vi "FieldPlaneRotation.vi"(8 "Bv (T)":dbl, 9 "Bu (T)":dbl, 10 "AlfaY (rad)":dbl, 11 "AlfaX (rad)":dbl) -> (1 "Bz (T)":dbl, 2 "By (T)":dbl, 3 "Bx (T)":dbl)   [LabVIEW 2020]
uses:
  <vilib>/imath/engines/lvmath2/RunTimeEngine/ArithmeticOperatorToken/NIMS_ArithmeticOperator_multmx-internal.vi
  <instcachedir>/0/NIMS_ArithmeticOperator_multmx-internal_B44B9A6937C8407A9A8862E3F2935EB3.lvgen/NIMS_ArithmeticOperator_multmx-internal_B44B9A6937C8407A9A8862E3F2935EB3_004.vi
  <vilib>/imathl/engines/lvmath/Functions/Error Handling/Create Error.vi
  <vilib>/imath/engines/lvmath2/RunTimeEngine/ArithmeticOperatorToken/NIMS_ArithmeticOperator_multmx(M,CV)-internal.vi
  <instcachedir>/0/NIMS_ArithmeticOperator_multmx(M,CV)-internal_19A14CC5BE0A4D31BE1E94A2E998D8C3.lvgen/NIMS_ArithmeticOperator_multmx(M,CV)-internal_19A14CC5BE0A4D31BE1E94A2E998D8C3_001.vi
  <vilib>/imath/engines/lvmath2/RunTimeEngine/IndexRead/NIMS V(S).vi
  <instcachedir>/0/NIMS V(S)_0488751826AF41519A22953C041130DC.lvgen/NIMS V(S)_0488751826AF41519A22953C041130DC_000.vi
  <vilib>/imath/engines/lvmath2/RunTimeEngine/NodeEndStatement/NIMS_NodeEndStatement_Output.vi
  <instcachedir>/0/NIMS_NodeEndStatement_Output_53EC0D466D134D7ABD903AC30B43404B.lvgen/NIMS_NodeEndStatement_Output_53EC0D466D134D7ABD903AC30B43404B_001.vi
  <vilib>/imath/engines/lvmath2/RunTimeEngine/ErrorHandling/NIMS_Finalize Error.vi
panel:
  # "Outputs"
  # "Inputs"
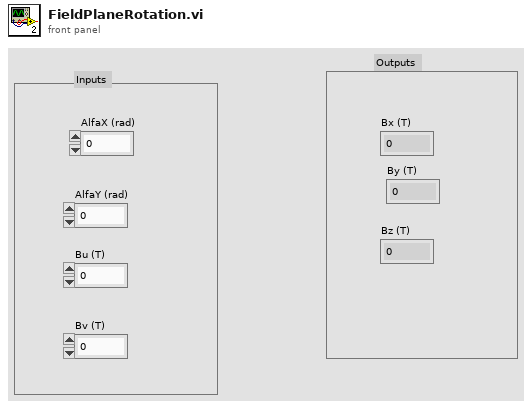
[diagram p1: front panel]
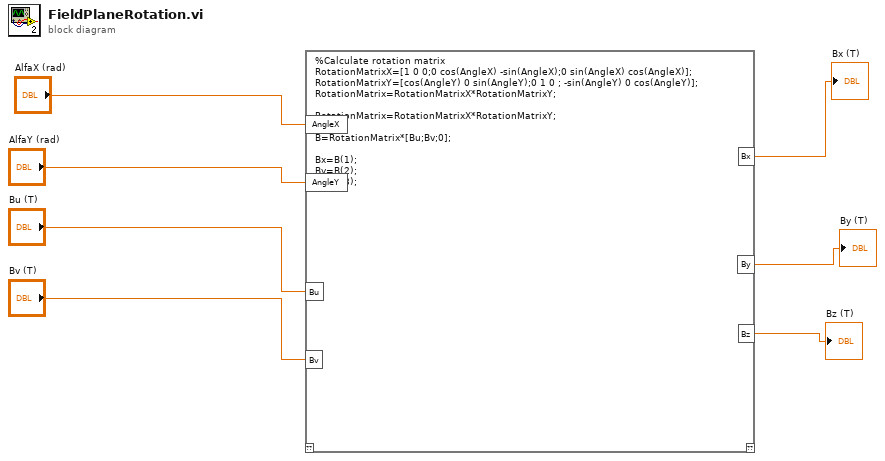
[diagram p0: block diagram]
diagram:
  n1 = mathscript code="%Calculate rotation matrix\nRotationMatrixX=[1 0 0;0 cos(AngleX) -sin(AngleX);0 sin(AngleX) cos(AngleX)];\nRotationMatrixY=[cos(AngleY) 0 sin(AngleY);0 1 0 ; -sin(AngleY) 0 cos(AngleY)];\nRotationMatrix=RotationMatrixX*RotationMatrixY;\n\nRotationMatrix=RotationMatrixX*RotationMatrixY;\n    \nB=RotationMatrix*[Bu;Bv;0];\n\nBx=B(1);\nBy=B(2);\nBz=B(3);"("AngleX"="AlfaX (rad)", "AngleY"="AlfaY (rad)", "Bu"="Bu (T)", "Bv"="Bv (T)") -> ("Bx"=→"Bx (T)":dbl, "By"=→"By (T)":dbl, "Bz"=→"Bz (T)":dbl)  [unwired: 1 in, 1 out]
